vi "AlliGator Update Channel File Settings.vi"(8 "Error In":errorcluster, 9 "Channel Arithmetic":T1, 10 "Selected Channel Name":string, 11 "Available Channel Names":string[](array[string])) -> (0 "Error Out":errorcluster)   [LabVIEW 2021, in "AlliGator Settings.lvlib"]
doc: "Updates the values of the <B>Channel Name</b> and <B>Channel Arithmetic</b> controls, as well as of the hidden <B>Available Channel Names</b> indicator."
uses:
  AlliGator Settings.lvlib
  AlliGator Gate Arithmetic.ctl
  AlliGator Settings Event.ctl
  AlliGator Settings Window Messages.ctl
  Dual-Channel Datasets/AlliGator Dual-Channel Datasets.lvlib
panel:
  # "see the AlliGator License on the block diagram (Ctrl+E or Window:Show Block Diagram)"
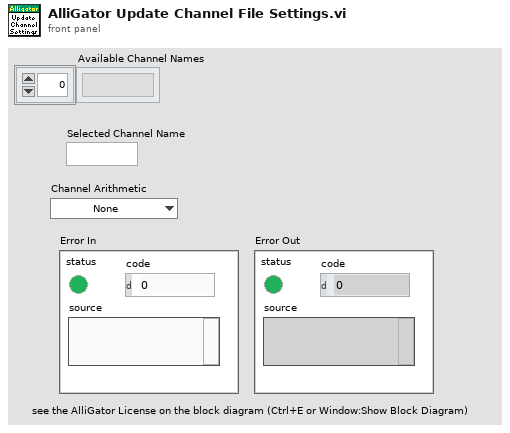
[diagram p1: front panel]
types:
  T1 = typedef "AlliGator Settings.lvlib/AlliGator Gate Arithmetic.ctl" = enum16{"None", "INT-G2", "G2/INT*<INT>", "(1 - G2/INT)*<INT>"}
  T2 = typedef "AlliGator Settings.lvlib/AlliGator Settings Event.ctl" = cluster{"AlliGator Settings Message":T3, "Sender":string, "Control Label":string, "Data":variant}
  T3 = typedef "AlliGator Settings.lvlib/AlliGator Settings Window Messages.ctl" = enum16{"Idle", "Subscribe", "Unsubscribe", "Refresh Parameter", "Refresh All Parameters", "Quit"}
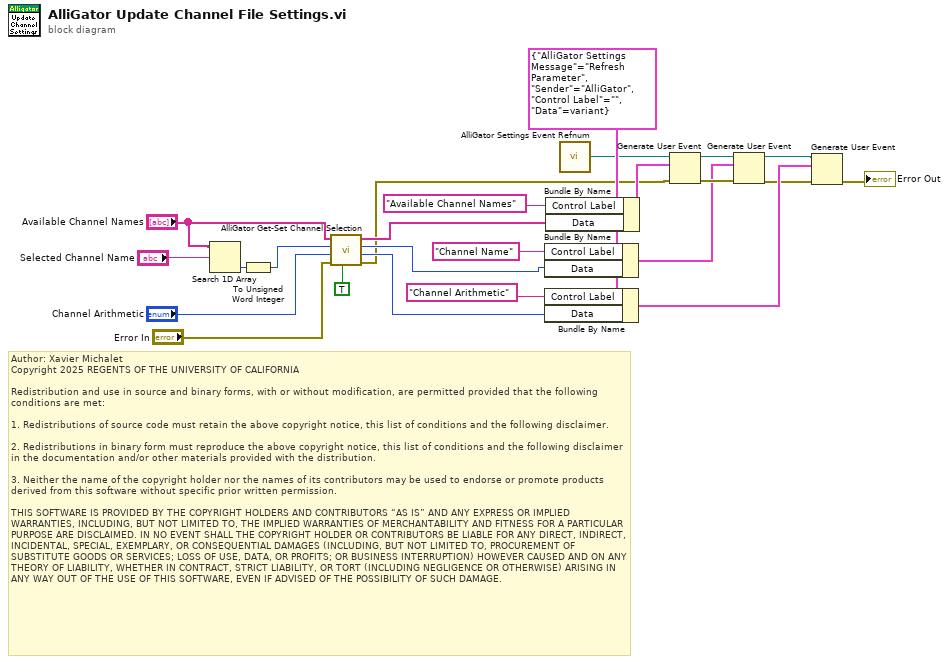
[diagram p0: block diagram]
diagram:
  w18 = T2 {"AlliGator Settings Message"=enum."Refresh Parameter", "Sender"="AlliGator", "Control Label"="", "Data"=variant} ("event data")
  # "Author: Xavier Michalet\nCopyright 2025 REGENTS OF THE UNIVERSITY OF CALIFORNIA\n\nRedistribution and use in source and binary forms, with or without modification, are permitted provided that the following conditions are met:\n\n1. Redistributions of source code must retain the above copyright notice, this list of conditions and the following disclaimer.\n\n2. Redistributions in binary form must reproduce the above copyright notice, this list of conditions and the following disclaimer in the documentation and/or other materials provided with the distribution.\n\n3. Neither the name of the copyright holder nor the names of its contributors may be used to endorse or promote products derived from this software without specific prior written permission.\n\nTHIS SOFTWARE IS PROVIDED BY THE COPYRIGHT HOLDERS AND CONTRIBUTORS “AS IS” AND ANY EXPRESS OR IMPLIED WARRANTIES, INCLUDING, BUT NOT LIMITED TO, THE IMPLIED WARRANTIES OF MERCHANTABILITY AND FITNESS FOR A PARTICULAR PURPOSE ARE DISCLAIMED. IN NO EVENT SHALL THE COPYRIGHT HOLDER OR CONTRIBUTORS BE LIABLE FOR ANY DIRECT, INDIRECT, INCIDENTAL, SPECIAL, EXEMPLARY, OR CONSEQUENTIAL DAMAGES (INCLUDING, BUT NOT LIMITED TO, PROCUREMENT OF SUBSTITUTE GOODS OR SERVICES; LOSS OF USE, DATA, OR PROFITS; OR BUSINESS INTERRUPTION) HOWEVER CAUSED AND ON ANY THEORY OF LIABILITY, WHETHER IN CONTRACT, STRICT LIABILITY, OR TORT (INCLUDING NEGLIGENCE OR OTHERWISE) ARISING IN ANY WAY OUT OF THE USE OF THIS SOFTWARE, EVEN IF ADVISED OF THE POSSIBILITY OF SUCH DAMAGE."
  n1 = Search 1D Array(1D array="Available Channel Names", element="Selected Channel Name") -> (index of element=w9:i32)  [unwired: 1 in]
  n2 = To Unsigned Word Integer(number=w9) -> (unsigned 16bit integer=w6:u16)
  n3 = call "AlliGator Get-Set Channel Selection.vi"("Set (T)/Get (F)"=TRUE, "error in (no error)"="Error In", "Channel Arithmetic"="Channel Arithmetic", "Selected Channel Name"=w6, "Available Channel Names"="Available Channel Names") -> ("error out"=w2:errorcluster, "Channel Arithmetic"=w3:T1, "Selected Channel Name"=w5:u16, "Available Channel Names"=w7:string[])  [unwired: 3 in]
  n4 = Bundle By Name(cluster=w18, "Control Label"="Channel Name", "Data"=w5) -> (w16:T2)
  n5 = Bundle By Name(cluster=w18, "Control Label"="Channel Arithmetic", "Data"=w3) -> (w21:T2)
  n6 = Bundle By Name(cluster=w18, "Control Label"="Available Channel Names", "Data"=w7) -> (w14:T2)
  n7 = call "AlliGator Settings Event Refnum.vi"() -> ("AlliGator Settings Event Refnum"=w13:refnum<user-event>)  [unwired: 8 in, 1 out]
  n8 = Generate User Event(user event=w13, event data cluster=w14, error in=w2) -> (user event out=w15:refnum<user-event>, error out=w17:errorcluster)  [unwired: 1 in]
  n9 = Generate User Event(user event=w15, event data cluster=w16, error in=w17) -> (user event out=w19:refnum<user-event>, error out=w20:errorcluster)  [unwired: 1 in]
  n10 = Generate User Event(user event=w19, event data cluster=w21, error in=w20) -> (error out=→"Error Out":errorcluster)  [unwired: 1 in, 1 out]
